vi "SetupGazeboGlobals.vi"   [LabVIEW 2012]
uses:
  <userlib>/rosforlv/ROS/Code/_ROSDefinition.vi
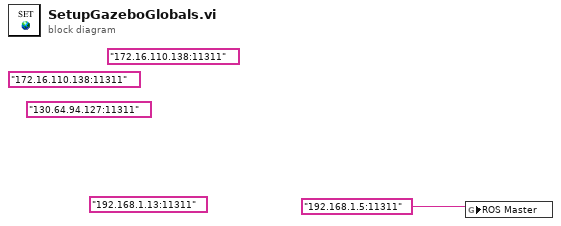
[diagram p0: block diagram]
diagram:
  (unwired) "192.168.1.13:11311" ("ROS Master")
  (unwired) "172.16.110.138:11311" ("ROS Master")
  (unwired) "130.64.94.127:11311" ("ROS Master")
  (unwired) "172.16.110.138:11311" ("ROS Master")
  n1 = global write "_ROSDefinition.vi" "ROS Master"("192.168.1.5:11311" ("ROS Master")) -> ()
